vi "Set Settings.vi"(8 "error in (no error)":errorcluster, 10 "component settings":T1[](array[typedef]), 11 "Component Settings Editor in":refnum<class "Component Settings Editor.lvclass">) -> (0 "error out":errorcluster, 3 "Component Settings Editor out":refnum<class "Component Settings Editor.lvclass">)   [LabVIEW 2019, in "DSF Core.lvlib" / "Component Settings Editor.lvclass"]
uses:
  Component Settings Editor.lvclass
  Typedefs/DSF Settings Info.ctl
  Component Settings Editor.lvclass/Component Settings Editor.ctl
  User Interface.lvclass
  DSF Core.lvlib
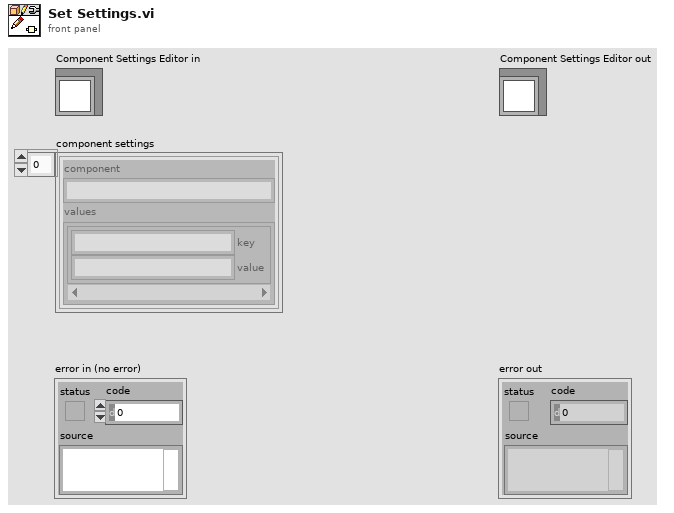
[diagram p1: front panel]
types:
  T1 = typedef "DSF Core.lvlib/DSF Settings Info.ctl" = cluster{"component":string, "values":cluster{"key":string, "value":string}[]}
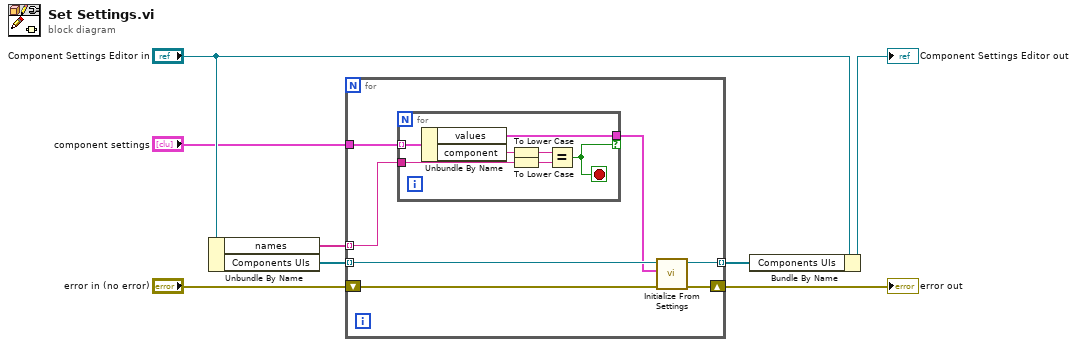
[diagram p0: block diagram]
diagram:
  n1 = Unbundle By Name("Component Settings Editor in") -> ("names"=w2:string[], "Components UIs"=w3:refnum<class "User Interface.lvclass">[])
  n2 = for {
    tunnel: [w15] -> w5 mode=indexing
    shift-right: [w14] -> w6
    shift-left: "error in (no error)" -> [w11]
    tunnel: "component settings" -> [w13]
    tunnel: w3 -> [w10] mode=indexing
    tunnel: w2 -> [w12] mode=indexing
    n3 = for {
      tunnel: w13 -> [w22] mode=indexing
      tunnel: w12 -> [w21]
      tunnel: [w20] -> w9 if=w19
      stop <- w19 stop-if-true
      n4 = Unbundle By Name(w22) -> ("values"=w20:cluster{"key":string, "value":string}[], "component"=w18:string)
      n5 = To Lower Case(string=w18) -> (all lower case string=w16:string)
      n6 = To Lower Case(string=w21) -> (all lower case string=w17:string)
      n7 = Equal?(x=w16, y=w17) -> (x = y?=w19:bool)
    }
    n8 = call "Initialize From Settings.vi"("error in (no error)"=w11, "settings"=w9, "User Interface in"=w10) -> ("error out"=w14:errorcluster, "User Interface out"=w15:refnum<class "User Interface.lvclass">)  [unwired: 7 in]
  }
  "error out" <- w6
  n9 = Bundle By Name(cluster="Component Settings Editor in", "Components UIs"=w5) -> (→"Component Settings Editor out":refnum<class "Component Settings Editor.lvclass">)
